vi "10-Tap 8-Bit Camera with DRAM (Host).vi"() -> ()   [LabVIEW 2014]
doc: "This is the host VI for the 10-Tap 8-Bit Camera with DRAM example. This example demonstrates how to acquire images from a 10-tap, 8-bit, extended configuration, Camera Link camera and display the images on the host. This example supports area scan and line scan cameras for both continuous and finite acquisitions.\n\nThis example also demonstrates the use of DRAM as a frame buffer for very high speed acquisitions. Data packing and flow-control are also employed to maximize use of the available DRAM and FIFOs in terms of both memory space and performance.\n\nAdditionally, the example demonstrates the serial server, which allows third-party camera configuration utilities to communicate with the camera using the Camera Link serial interface while this VI is running."
uses:
  <vilib>/userdefined/High Color/nirio_resource_hc.ctl
  <vilib>/FPGAPlugInAG/PCIe-1473R/niLvFpga_Open_PCIe-1473R.vi
  <vilib>/rvi/interface/common/dynamic/niFpgaDynamicAddResources.vi
  <vilib>/FPGAPlugInAG/Dynamic/niLvFpga_Reset_Dynamic.vi
  <vilib>/Utility/error.llb/Error Cluster From Error Code.vi
  <vilib>/rvi/errors/niLvFpgaAdjustHostInterfaceError.vi
  <vilib>/FPGAPlugInAG/Dynamic/niLvFpga_Run_Dynamic.vi
  <vilib>/rvi/interface/common/niFpgaWaitOnOcc.vi
  <vilib>/DAQmx/write.llb/DAQmx Write (Analog DBL 1Chan 1Samp).vi
  <vilib>/FPGAPlugInAG/Dynamic/niLvFpga_Close_Dynamic.vi
  <vilib>/rvi/interface/nirviOpenFPGA/nirviOpenFPGA.xnode
  FPGA Bitfiles/10-Tap8-bitCamer_FPGATarget_10-Tap8-bitCamer_C490DC32.lvbitx
  10-Tap 8-Bit Camera with DRAM (FPGA).vi
  <vilib>/rvi/interface/nirviMethod/nirviMethod.xnode
  <vilib>/rvi/interface/nirviReadWriteControl/nirviReadWriteControl.xnode
  <vilib>/rvi/interface/nirviCloseFPGA/nirviCloseFPGA.xnode
  <vilib>/rvi/interface/Simulation/niFpgaSimulationCallBeginRW.vi
  <vilib>/rvi/errors/niLvFpgaMergeErrorWithErrorCode.vi
  NiFpgaLv.dll
  <vilib>/FPGAPlugInAG/Dynamic/niLvFpga_ConfigureFifo_Dynamic.vi
  <vilib>/FPGAPlugInAG/Dynamic/niLvFpga_StartFifo_Dynamic.vi
  <vilib>/FPGAPlugInAG/Dynamic/niLvFpga_ReadFifo_Dynamic.vi
  fish tracking dll/labview/find_fish_position.lvlib
  fish tracking dll/bin/find_fish_position.dll
panel:
  in  "shift":i32=10
  in  "ROI_height":i32=300
  in  "ROI_witdth":i32=300
  out "Centroid":cluster{"y":i32, "x":i32}
  in  "SpeedFactor":dbl=1.0
  in  "offset":dbl(slide)=179.73568281938327 scale=150.0..250.0
  in  "Y_Target":dbl=384.0
  in  "X_Target":dbl=520.0
  out "TimeDelay":dbl
  in  "setROI":bool
  out "DstImageOpenCV":T1(plugin-control)
  in  "Esize_open":i32(slide)=4 scale=0.0..10.0
  in  "Esize_close":i32(slide)=4 scale=0.0..10.0
  in  "BinThreshold":i32(slide)=118 scale=0.0..255.0
  in  "DMA Buffer Size\n(In Images)":u32=64 caption="DMA Buffer Size"
  in  "Signal Mapping":T2(ring)=enum."Basler 10-tap"
  out "Acq In Progress":bool
  in  "Line Scan":bool
  in  "Frames To Acquire":u32 caption="Frames To Acquire\n(0 = infinite)"
  in  "Cancel":bool
  out "Acq'd Frame Width":u32
  in  "Stopped":bool
  in  "RIO Device":T3="Horizontal"
  out "DMA Write Timeout":bool
  in  "Start Serial Server":bool=TRUE
  out "Frames Acq'd":u32
  out "Acq'd Frame Height":u32
  out "Image":T1(plugin-control)
  in  "Acquire":bool
  in  "Stop":bool
  in  "Image Height":u32=768 max=65535
  in  "Image Width":u32=1040 max=65535 step=40
  out "Initialized":bool
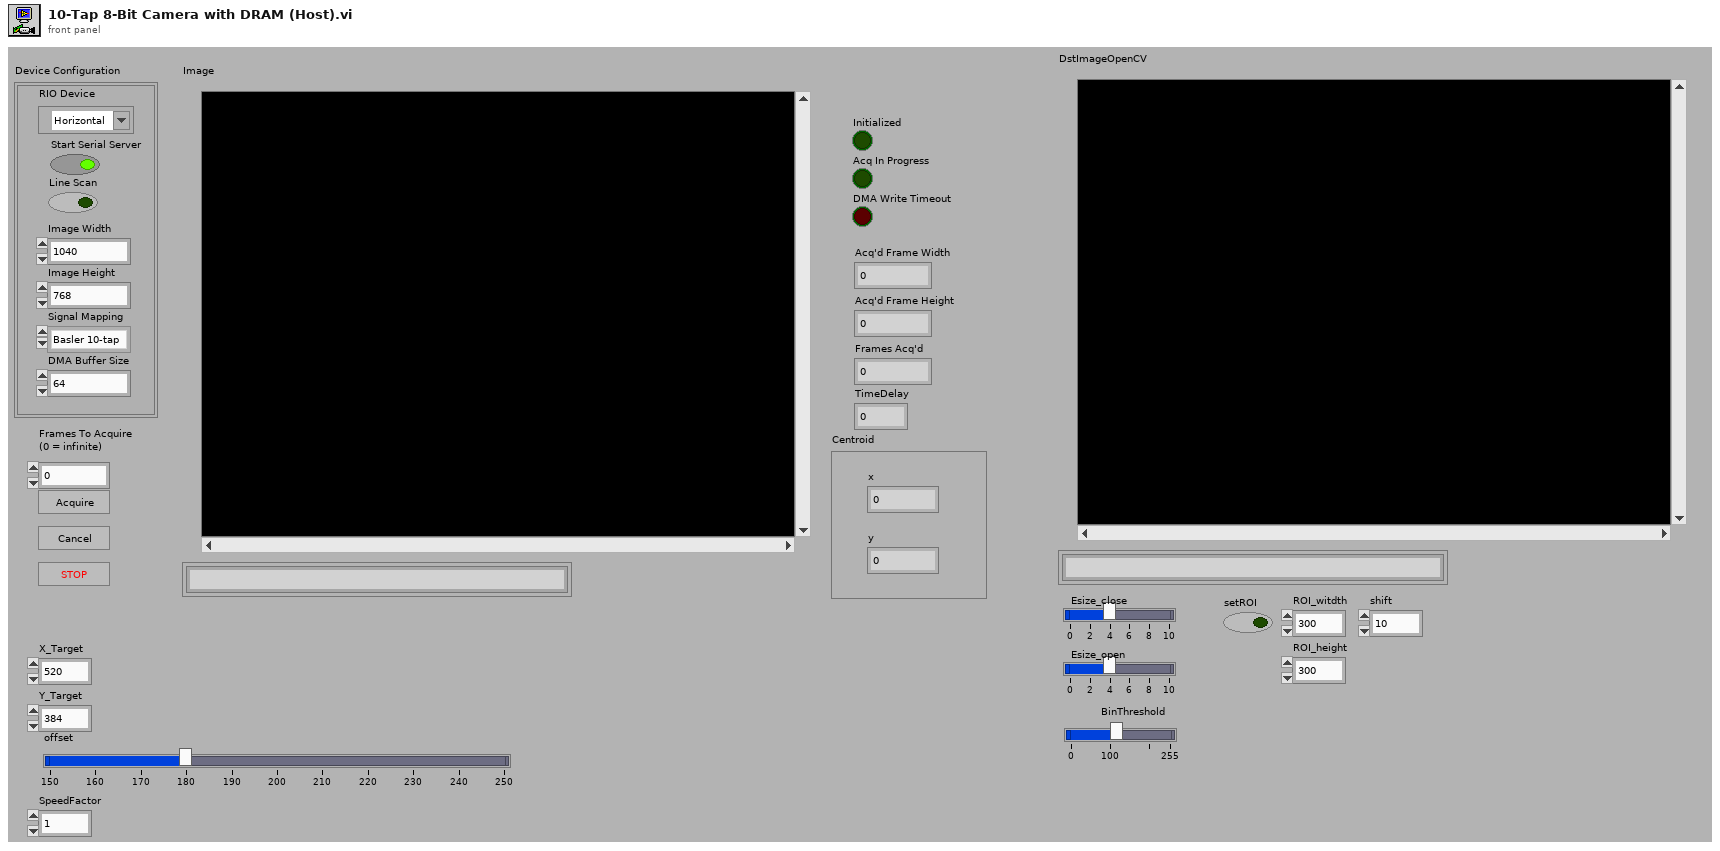
[diagram p1: front panel]
types:
  T1 = typedef "IMAQ Image.ctl" = refnum<image>
  T2 = enum8{"Standard", "Basler 10-tap", "Vosskühler 10-tap"}
  T3 = typedef "nirio_resource_hc.ctl" = tag
  T4 = typedef "Image Type" = u32
  T5 = enum16{"big-endian, network order", "native, host order", "little-endian"}
  T6 = enum32{"Map Pixel Pointer", "Unmap Pixel Pointer", "Get Pixels Infos"}
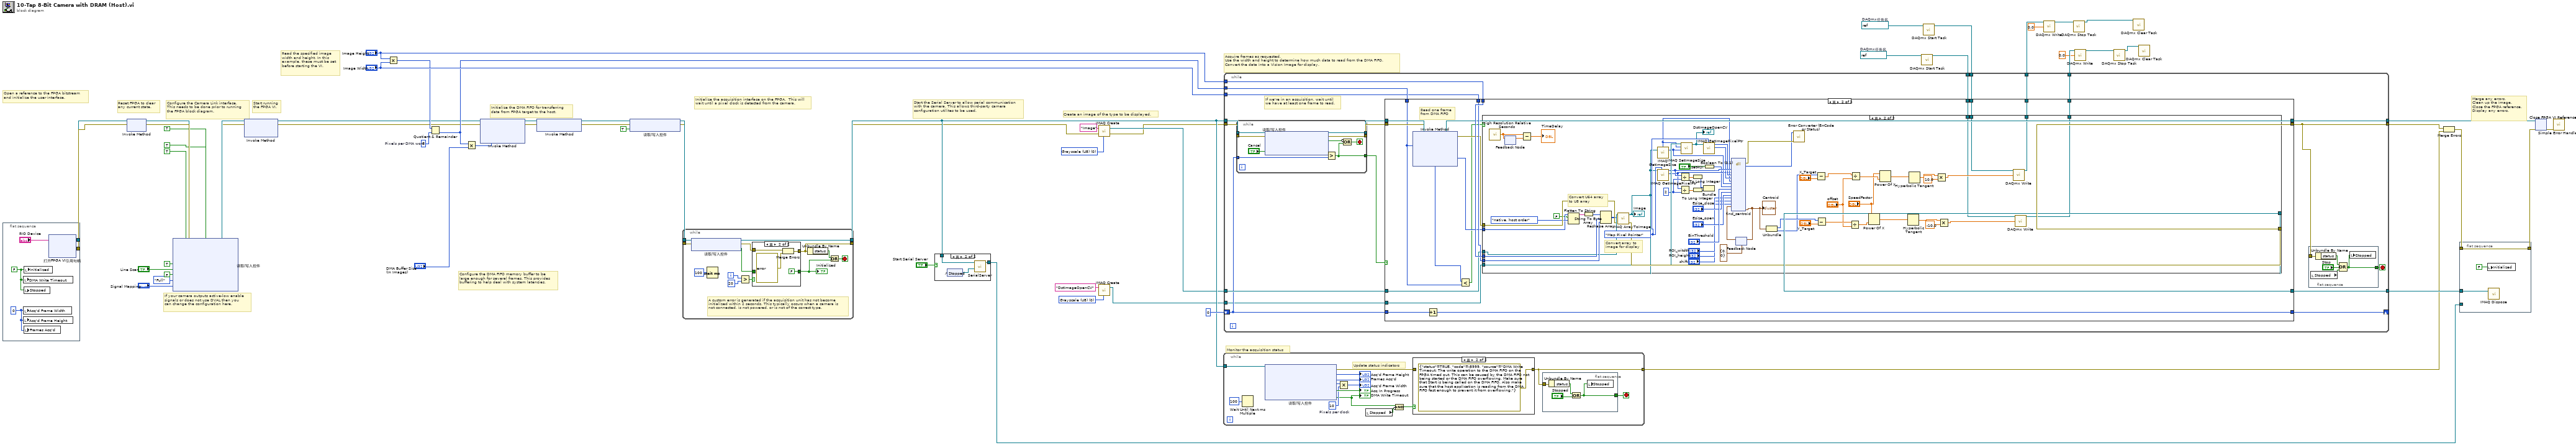
[diagram p0: block diagram]
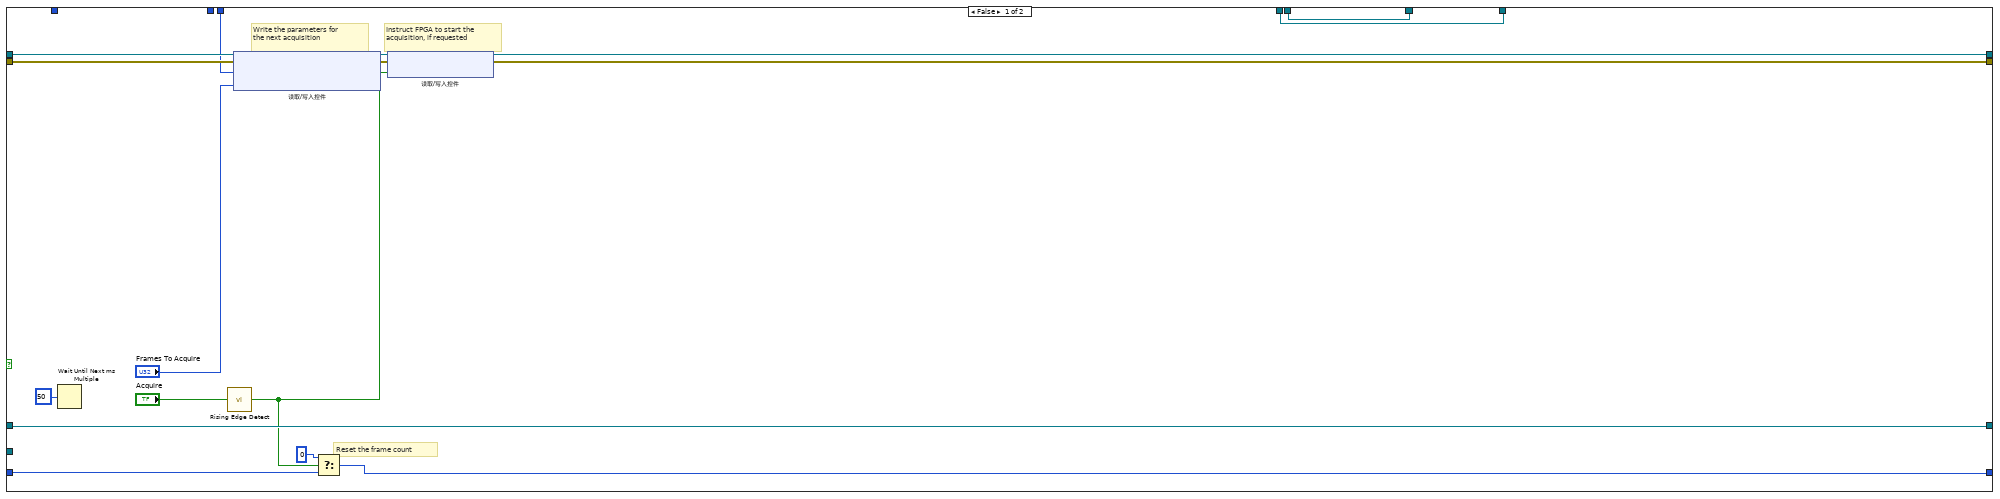
[diagram p4: hidden frame]
diagram:
  w11 = refnum<k21> "Stage_Y"  # DAQmx任务名
  w12 = refnum<k21> "Stage_X"  # DAQmx任务名
  w14 = T4 0 items=["Grayscale (U8)", "Grayscale (I16)", "Grayscale (SGL)", "Complex (CSG)", "RGB (U32)", "HSL (U32)", "RGB (U64)", "Grayscale (U16)"] ("Image Type")
  w20 = u32 8  # Pixels per DMA word
  w57 = T4 0 items=["Grayscale (U8)", "Grayscale (I16)", "Grayscale (SGL)", "Complex (CSG)", "RGB (U32)", "HSL (U32)", "RGB (U64)", "Grayscale (U16)"] ("Image Type")
  # "If your camera outputs active-low enable\nsignals or does not use DVAL then you \ncan change the configuration here."
  # "Configure the DMA FIFO memory buffer to be\nlarge enough for several frames. This provides\nbuffering to help deal with system latencies."
  # "Start running\nthe FPGA VI."
  # "Reset FPGA to clear\nany current state."
  # "Read the specified image\nwidth and height. In this\nexample, these must be set\nbefore starting the VI."
  # "Merge any errors.\nClean up the image.\nClose the FPGA reference.\nDisplay any errors."
  # "Acquire frames as requested.\nUse the width and height to determine how much data to read from the DMA FIFO.\nConvert the data into a Vision Image for display."
  # "Monitor the acquisition status"
  # "Start the Serial Server to allow serial communication\nwith the camera. This allows third-party camera\nconfiguration utilites to be used."
  # "Create an image of the type to be displayed."
  # "Initialize the acquisition interface on the FPGA.  This will\nwait until a pixel clock is detected from the camera."
  # "Initialize the DMA FIFO for transferring\ndata from FPGA target to the host."
  # "Configure the Camera Link interface.\nThis needs to be done prior to running\nthe FPGA block diagram."
  # "Open a reference to the FPGA bitstream\nand initialize the user interface."
  n1 = flat-sequence {
    tunnel: [w63] -> w48
    tunnel: [w62] -> w61
    frame #0 {
      w66 = u32 0 ("Num Lines Acq'd")
      w65 = FALSE ("stop")
      n2 = local write "DMA Write Timeout"(w65) -> ()
      n3 = local write "Acq'd Frame Width"(w66) -> ()
      n4 = local write "Acq'd Frame Height"(w66) -> ()
      n5 = local write "Stopped"(w65) -> ()
      n6 = local write "Frames Acq'd"(w66) -> ()
      n7 = local write "Initialized"(w65) -> ()
      n8 = xnode "打开FPGA VI引用句柄"("资源名称"="RIO Device") -> ("FPGA VI引用输出"=w63:refnum<k20>, "错误输出"=w62:errorcluster)  [unwired: 1 in]
    }
  }
  n9 = xnode "Invoke Method"("FPGA VI引用输入"=w48, "错误输入"=w61) -> ("FPGA VI引用输出"=w37:refnum<k20>, "错误输出"=w40:errorcluster)
  n10 = xnode "读取/写入控件"("FPGA VI引用输入"=w37, "错误输入"=w40, "CL Config.FVAL Active High"=TRUE ("IO Module Config.CL FVAL Active High"), "CL Config.LVAL Active High"=TRUE ("IO Module Config.CL LVAL Active High"), "CL Config.DVAL Active High"=TRUE ("IO Module Config.CL DVAL Active High"), "CL Config.Spare Active High"=TRUE ("IO Module Config.CL Spare Active High"), "CL Config.Line Scan"="Line Scan", "Acq Control.Ignore DVAL"=FALSE ("CL Config.Line Scan"), "CL Config.Configuration"=enum8{"Base", "Medium", "Full"}."Full", "CL Config.Signal Mapping"="Signal Mapping") -> ("FPGA VI引用输出"=w41:refnum<k20>, "错误输出"=w39:errorcluster)
  n11 = xnode "Invoke Method"("FPGA VI引用输入"=w41, "错误输入"=w39) -> ("FPGA VI引用输出"=w17:refnum<k20>, "错误输出"=w16:errorcluster)  [unwired: 1 in]
  n12 = Multiply(x="Image Height", y="Image Width") -> (x*y=w19:u32)
  n13 = Quotient & Remainder(x=w19, y=w20) -> (floor(x/y)=w18:u32)  [unwired: 1 out]
  n14 = Multiply(x=w18, y="DMA Buffer Size\n(In Images)") -> (x*y=w31:u32)
  n15 = xnode "Invoke Method"("FPGA VI引用输入"=w17, "错误输入"=w16, "请求的深度"=w31) -> ("FPGA VI引用输出"=w47:refnum<k20>, "错误输出"=w46:errorcluster)  [unwired: 1 out]
  n16 = xnode "Invoke Method"("FPGA VI引用输入"=w47, "错误输入"=w46) -> ("FPGA VI引用输出"=w32:refnum<k20>, "错误输出"=w45:errorcluster)
  n17 = xnode "读取/写入控件"("FPGA VI引用输入"=w32, "错误输入"=w45, "Acq Control.Initialize"=TRUE ("Arm Acquisition")) -> ("FPGA VI引用输出"=w60:refnum<k20>, "错误输出"=w59:errorcluster)
  n18 = while {
    tunnel: w60 -> [w74]
    tunnel: w59 -> [w73]
    tunnel: [w72] -> w28
    tunnel: [w76] -> w27
    i -> [w68]
    stop <- w79 stop-if-true
    # "A custom error is generated if the acquisition unit has not become\ninitialized within 2 seconds. This typically occurs when a camera is\nnot connected, is not powered, or is not of the correct type."
    n19 = xnode "读取/写入控件"("FPGA VI引用输入"=w74, "错误输入"=w73) -> ("FPGA VI引用输出"=w72:refnum<k20>, "错误输出"=w71:errorcluster, "Acq Status.Initialized"=w70:bool)
    n20 = Wait (ms)(milliseconds to wait=u32 100) -> ()  [unwired: 1 out]
    n21 = Greater?(x=w68, y=20) -> (0:w69:bool)
    n22 = case shown="真" w69 {
      tunnel: [w81 FALSE] -> w75
      tunnel: w70 -> [w81 _]
      tunnel: w71 -> [w80 w83]
      tunnel: [w80 w85] -> w76
      frame False {
      }
      frame True {
        n23 = Merge Errors(w83, errorcluster {"status"=TRUE, "code"=-8999, "source"="Acquisition Initialization: This error typically occurs when a camera is not properly connected, is not powered, or is not of the correct type."} ("error in")) -> (w85:errorcluster)
      }
    }
    "Initialized" <- w75
    n24 = Unbundle By Name(w76) -> ("status"=w78:bool)
    n25 = Or(x=w78, y=w75) -> (x .or. y?=w79:bool)
  }
  n26 = case shown="真" "Start Serial Server" {
    tunnel: [_ w86] -> w49
    tunnel: w28 -> [_ w87]
    frame False {
    }
    frame True {
      n27 = control-ref of="Stopped"() -> (w88:refnum<vi>)
      n28 = call "SerialServer.vi"("Stop Refnum"=w88, "FPGA VI Reference In"=w87) -> ("FPGA VI Reference Out"=w86:refnum<k20>)  [unwired: 5 in]
    }
  }
  n29 = call "IMAQ Create"("Image Name"="Image", "Image Type"=w57, "error in (no error)"=w27) -> ("New Image"=w24:T1, "error out"=w23:errorcluster)  [unwired: 2 in]
  n30 = call "IMAQ Create"("Image Name"="DstImageOpenCV", "Image Type"=w14) -> ("New Image"=w13:T1)  [unwired: 3 in, 1 out]
  n31 = while {
    tunnel: w28 -> [w99]
    tunnel: [w102] -> w42
    stop <- w101 stop-if-true
    w92 = u32 10  # Pixels per clock
    # "Update status indicators"
    n32 = Wait Until Next ms Multiple(millisecond multiple=u32 100) -> ()  [unwired: 1 out]
    n33 = xnode "读取/写入控件"("FPGA VI引用输入"=w99) -> ("错误输出"=w98:errorcluster, "Acq Status.Lines Per Frame"=→"Acq'd Frame Height":u32, "Acq Status.Frames Acq'd"=→"Frames Acq'd":u32, "Acq Status.Clocks Per Line"=w93:u32, "Acq Status.Acq In Progress"=→"Acq In Progress":bool, "Acq Status.DMA Write Timeout"=w90:bool)  [unwired: 1 in, 1 out]
    "DMA Write Timeout" <- w90
    n34 = Multiply(x=w93, y=w92) -> (x*y=→"Acq'd Frame Width":u32)
    n35 = local read "Stopped"() -> (w89:bool)
    n36 = Compound Arithmetic op=AND(w90, invert w89) -> (w91:bool)
    n37 = case shown="真" w91 {
      tunnel: w98 -> [w107 _]
      tunnel: [w107 errorcluster {"status"=TRUE, "code"=-8999, "source"="DMA Write Timeout: The write operation to the DMA FIFO on the FPGA timed out. This can be caused by the DMA FIFO not being started or the DMA FIFO overflowing. Make sure that Start is being called on the DMA FIFO. Also make sure that the host application is reading from the DMA FIFO fast enough to prevent it from overflowing."} ("error out")] -> w102
      frame False {
      }
      frame True {
      }
    }
    n38 = flat-sequence {
      tunnel: w102 -> [w106]
      tunnel: [w104] -> w101
      frame #0 {
        n39 = Unbundle By Name(w106) -> ("status"=w105:bool)
        n40 = Or(x=w105, y="Stopped") -> (x .or. y?=w104:bool)
        n41 = local write "Stopped"(w104) -> ()
      }
    }
  }
  n42 = call <vilib>:"DAQmx Start Task.vi"("task/channels in"=w11) -> ("task out"=w9:refnum<k21>)  [unwired: 13 in, 1 out]
  n43 = call <vilib>:"DAQmx Start Task.vi"("task/channels in"=w12) -> ("task out"=w10:refnum<k21>)  [unwired: 13 in, 1 out]
  n44 = while {
    tunnel: w28 -> [w120]
    tunnel: w23 -> [w119]
    tunnel: w18 -> [w128]
    tunnel: "Image Height" -> [w127]
    tunnel: "Image Width" -> [w126]
    tunnel: w24 -> [w125]
    tunnel: [w123] -> w43
    tunnel: [w124] -> w56
    tunnel: [w121] -> w51
    shift-right: [w115] -> _
    shift-left: u32 0 -> [w114]
    tunnel: w13 -> [w113]
    tunnel: w10 -> [w112]
    tunnel: w9 -> [w111]
    tunnel: [w110] -> w8
    tunnel: [w109] -> w7
    stop <- w122 stop-if-true
    # "If we're in an acquisition, wait until\nwe have at least one frame to read."
    n45 = while {
      tunnel: w120 -> [w135]
      tunnel: w119 -> [w134]
      tunnel: [w132] -> w118
      tunnel: [w133] -> w117
      tunnel: w114 -> [w138]
      tunnel: [w136] -> w116
      stop <- w137 stop-if-true
      n46 = xnode "读取/写入控件"("FPGA VI引用输入"=w135, "错误输入"=w134, "Acq Control.Cancel Acq"="Cancel") -> ("FPGA VI引用输出"=w133:refnum<k20>, "错误输出"=w132:errorcluster, "Acq Status.Acq In Progress"=w131:bool, "Acq Status.Frames Acq'd"=w130:u32)
      n47 = Greater?(x=w130, y=w138) -> (0:w136:bool)
      n48 = Compound Arithmetic op=OR(invert w131, w136) -> (w137:bool)
    }
    n49 = case shown="真" w116 {
      tunnel: w117 -> [w156 w173]
      tunnel: w118 -> [w155 w172]
      tunnel: w128 -> [_ w166]
      tunnel: w127 -> [w149 w180]
      tunnel: w126 -> [_ w179]
      tunnel: w125 -> [w160 w178]
      tunnel: [w151 w176] -> w123
      tunnel: [w154 w175] -> w124
      tunnel: [w160 w174] -> w121
      tunnel: w114 -> [w157 w171]
      tunnel: [w159 w170] -> w115
      tunnel: w113 -> [_ w165]
      tunnel: w112 -> [w145 w164]
      tunnel: w111 -> [w144 w163]
      tunnel: [w145 w162] -> w110
      tunnel: [w144 w161] -> w109
      frame False {
        # "Reset the frame count"
        # "Instruct FPGA to start the\nacquisition, if requested"
        # "Write the parameters for\nthe next acquisition"
        n50 = Wait Until Next ms Multiple(millisecond multiple=u32 50) -> ()  [unwired: 1 out]
        n51 = call "Rising Edge Detect.vi"("Input"="Acquire") -> ("Pulse"=w146:bool)  [unwired: 4 in]
        n52 = xnode "读取/写入控件"("FPGA VI引用输入"=w156, "错误输入"=w155, "Acq Control.Line Scan Height"=w149, "Acq Control.Frames To Acq"="Frames To Acquire") -> ("FPGA VI引用输出"=w153:refnum<k20>, "错误输出"=w152:errorcluster)
        n53 = Select(t=u32 0, s=w146, f=w157) -> (s? t:f=w159:u32)
        n54 = xnode "读取/写入控件"("FPGA VI引用输入"=w153, "错误输入"=w152, "Acq Control.Acquire"=w146) -> ("FPGA VI引用输出"=w154:refnum<k20>, "错误输出"=w151:errorcluster)
      }
      frame True {
        # "Read one frame\nfrom DMA FIFO"
        n55 = xnode "Invoke Method"("FPGA VI引用输入"=w173, "错误输入"=w172, "元素数量"=w166) -> ("FPGA VI引用输出"=w175:refnum<k20>, "错误输出"=w177:errorcluster, "数据"=w169:u64[], "剩余元素"=w167:u32)  [unwired: 1 in]
        n56 = Increment(x=w171) -> (x+1=w170:u32)
        n57 = Less?(x=w167, y=w166) -> (x < y?=w168:bool)
        n58 = case shown="真" w168 {
          tunnel: w180 -> [_ w248]
          tunnel: w179 -> [_ w247]
          tunnel: w178 -> [w184 w246]
          tunnel: w177 -> [w183 w245]
          tunnel: [w183 w244] -> w176
          tunnel: [w184 w236] -> w174
          tunnel: w169 -> [_ w241]
          tunnel: w165 -> [_ w235]
          tunnel: w164 -> [w182 w200]
          tunnel: w163 -> [w181 w199]
          tunnel: [w182 w198] -> w162
          tunnel: [w181 w197] -> w161
          frame False {
            # "Do not display the image if we're falling behind in the acquisition."
          }
          frame True {
            w234 = u64 2 ("y")
            w237 = T6."Map Pixel Pointer" ("Function")
            # "Convert U64 array\nto U8 array"
            # "Convert array to\nimage for display"
            n59 = call <vilib>:"High Resolution Relative Seconds.vi"() -> ("relative seconds"=w218:dbl)
            n60 = feedback-in #1(w218) -> ()
            n61 = feedback #1() -> (w219:dbl)  [unwired: 1 in]
            n62 = Subtract(x=w218, y=w219) -> (x-y=→"TimeDelay":dbl)
            n63 = Flatten To String(anything=w241, prepend array or string size? (T)=FALSE, byte order (0:big-endian, network order)=T5."native, host order") -> (data string=w239:string)  [unwired: 1 in, 2 out]
            n64 = String To Byte Array(string=w239) -> (unsigned byte array=w238:u8[])
            n65 = Reshape Array(w238, w248, w247) -> (w243:u8[][])
            n66 = call "IMAQ ArrayToImage"("error in (no error)"=w245, "Image Pixels (U8)"=w243, "Image"=w246) -> ("error out"=w244:errorcluster, "Image Out"=w236:T1)  [unwired: 7 in]
            "Image" <- w236
            n67 = call "IMAQ GetImageSize"("Image"=w236) -> ("Y Resolution"=w226:i32, "X Resolution"=w227:i32)  [unwired: 3 in, 1 out]
            n68 = call "IMAQ GetImagePixelPtr"("Function"=w237, "Image"=w236) -> ("LineWidth(Pixels)"=w222:i32, "Pixel Pointer out"=w230:u64)  [unwired: 4 in, 4 out]
            n69 = Divide(x=w230, y=w234) -> (x/y=w233:dbl)
            n70 = Divide(x=w222, y=w234) -> (x/y=w232:dbl)
            n71 = call "IMAQ SetImageSize"("Y Resolution"=w226, "X Resolution"=w227, "Image"=w235) -> ("Image Out"=w231:T1)  [unwired: 2 in, 1 out]
            "DstImageOpenCV" <- w231
            n72 = To Long Integer(number=w233) -> (32bit integer=w196:i32)
            n73 = To Long Integer(number=w232) -> (32bit integer=w195:i32)
            n74 = call "IMAQ GetImagePixelPtr"("Function"=w237, "Image"=w231) -> ("LineWidth(Pixels)"=w228:i32, "Pixel Pointer out"=w229:u64)  [unwired: 4 in, 4 out]
            n75 = Boolean To (0,1)(Boolean="setROI") -> (0, 1=w221:i16)
            n76 = Bundle(w196, w195) -> ()  [unwired: 1 in, 1 out]
            n77 = feedback #2(cluster{"y":i32, "x":i32} {"y"=0, "x"=0} ("Centroid")) -> (w193:cluster{"y":i32, "x":i32})
            n78 = dll-call lib="C:/Users/Tracking/Documents/GitHub/Tracking/TrackingUsingOpenCV/fish tracking dll/bin/find_fish_position.dll" fn="find_centroid"("ImagePtrSrc"=w230, "LineWidthSrc"=w222, "ImagePtrDst"=w229, "LineWidthDst"=w228, "Width"=w227, "Height"=w226, "setROI"=w221, "BinThreshold"="BinThreshold", "Esize_close"="Esize_close", "Esize_open"="Esize_open", "ROI_witdth"="ROI_witdth", "ROI_height"="ROI_height", "shift"="shift", "centroid_in"=w193) -> (error out=w186:errorcluster, "return type"=w185:i32, "Centroid"=w194:cluster{"y":i32, "x":i32})  [unwired: 18 in, 1 out]
            "Centroid" <- w194
            n79 = feedback-in #2(w194) -> ()
            n80 = Unbundle(w194) -> ("y"=w188:i32, "x"=w187:i32)
            n81 = call "Error Converter (ErrCode or Status).vi"("error in (no error)"=w186, "error code"=w185) -> ()  [unwired: 9 in, 1 out]
            n82 = Subtract(x=w187, y="X_Target") -> (x-y=w214:dbl)
            n83 = Subtract(x=w188, y="Y_Target") -> (x-y=w213:dbl)
            n84 = Divide(x=w213, y="offset") -> (x/y=w210:dbl)
            n85 = Divide(x=w214, y="offset") -> (x/y=w211:dbl)
            n86 = Power Of X(1:w210, 2:"SpeedFactor") -> (0:w207:dbl)
            n87 = Power Of X(1:w211, 2:"SpeedFactor") -> (0:w208:dbl)
            n88 = Hyperbolic Tangent(1:w207) -> (0:w203:dbl)
            n89 = Hyperbolic Tangent(1:w208) -> (0:w204:dbl)
            n90 = Multiply(x=w204, y=10.0) -> (x*y=w202:dbl)
            n91 = Multiply(x=w203, y=-10.0) -> (x*y=w201:dbl)
            n92 = call-poly <vilib>:"DAQmx Write.vi"("task/channels in"=w200, "data"=w202) -> ("task out"=w198:refnum<k21>)  [unwired: 11 in, 2 out]
            n93 = call-poly <vilib>:"DAQmx Write.vi"("task/channels in"=w199, "data"=w201) -> ("task out"=w197:refnum<k21>)  [unwired: 11 in, 2 out]
          }
        }
      }
    }
    n94 = flat-sequence {
      tunnel: w123 -> [w141]
      tunnel: [w140] -> w122
      frame #0 {
        n95 = local read "Stopped"() -> (w139:bool)
        n96 = Unbundle By Name(w141) -> ("status"=w142:bool)
        n97 = Compound Arithmetic op=OR(w142, "Stop", w139) -> (w140:bool)
        n98 = local write "Stopped"(w140) -> ()
      }
    }
  }
  n99 = call-poly <vilib>:"DAQmx Write.vi"("task/channels in"=w8, "data"=0.0) -> ("task out"=w6:refnum<k21>)  [unwired: 11 in, 2 out]
  n100 = call <vilib>:"DAQmx Stop Task.vi"("task/channels in"=w6) -> ("task out"=w2:refnum<k21>)  [unwired: 13 in, 1 out]
  n101 = call-poly <vilib>:"DAQmx Write.vi"("task/channels in"=w7, "data"=0.0) -> ("task out"=w4:refnum<k21>)  [unwired: 11 in, 2 out]
  n102 = call <vilib>:"DAQmx Stop Task.vi"("task/channels in"=w4) -> ("task out"=w1:refnum<k21>)  [unwired: 13 in, 1 out]
  n103 = call <vilib>:"DAQmx Clear Task.vi"("task in"=w2) -> ()  [unwired: 14 in, 1 out]
  n104 = call <vilib>:"DAQmx Clear Task.vi"("task in"=w1) -> ()  [unwired: 14 in, 1 out]
  n105 = Merge Errors(w43, w42) -> (w44:errorcluster)
  n106 = flat-sequence {
    tunnel: w44 -> [w250]
    tunnel: [w250] -> w53
    tunnel: w51 -> [w251]
    tunnel: w49 -> [_]
    frame #0 {
      n107 = local write "Initialized"(FALSE ("Module Enabled")) -> ()
      n108 = call "IMAQ Dispose"("Image"=w251) -> ()  [unwired: 5 in, 1 out]
    }
  }
  n109 = xnode "Close FPGA VI Reference"("FPGA VI引用输入"=w56, "错误输入"=w53) -> ("错误输出"=w50:errorcluster)
  n110 = call <vilib>:"Simple Error Handler.vi"("error in (no error)"=w50) -> ()  [unwired: 4 in, 5 out]
